vi "LineDetection-2Steps.vi"() -> ()   [LabVIEW 2014]
doc: "This example shows how to use the Edge Tool in NI Vision. The Edge Tool finds edges (or sharp transitions in the pixels values) along a given line or ROI profile. The Edge Tool is a precursor function to many of the gauging and inspection tasks. For example, the location of the edges found along a line profile across an object can interpreted as the boundaries of the object whose dimensions have to be measured for a gauging application or the presence of a crack in the surface of an object for an inspection application."
uses:
  <vilib>/vision/NI_Vision_Development_Module.lvlib
panel:
  in  "Process":u16(ring)=2 items=["Get First Edge", "Get First + Last Edge", "Get All Edges", "Get Best Edge"]
  in  "Scan Direction":u16
  in  "Step Size":u32=5
  in  "Edge Options":T1={"Edge Polarity"=0, "Kernel Size"=3, "Width"=5, "Minimum Edge Strength"=10.0, "Interpolation Type"=1, "Data Processing Method"=0} {"Data Processing Method" items=["Average", "Median"]; "Interpolation Type" items=["Zero Order"=0, "Bilinear"=1, "Bilinear Fixed"=4]; "Minimum Edge Strength" min=0.0 max=255.0 format="%.2g"; "Width" min=1 step=2; "Kernel Size" min=3 step=2; "Edge Polarity" items=["All Edges", "Rising Edges", "Falling Edges"]}
  out "Image":T2(plugin-control)
  in  "Stop":bool
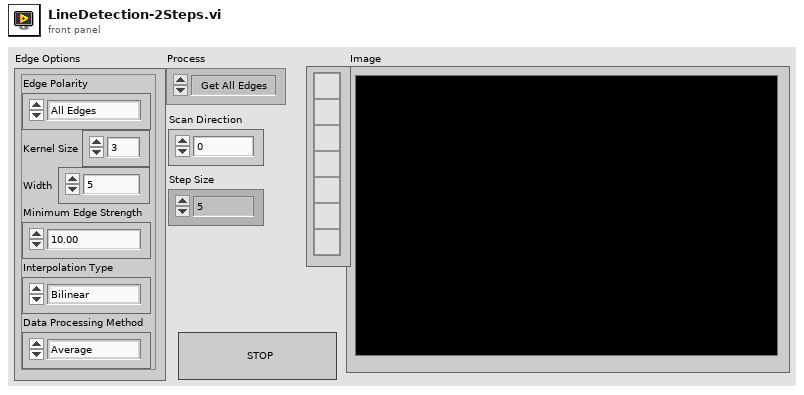
[diagram p1: front panel]
types:
  T1 = cluster{"Edge Polarity":u16, "Kernel Size":u32, "Width":u32, "Minimum Edge Strength":dbl, "Interpolation Type":u16, "Data Processing Method":u16}
  T2 = typedef "IMAQ Image.ctl" = refnum<image>
  T3 = typedef "IMAQ Circle" = cluster{"Center X":i32, "Center Y":i32, "Inner Radius":i32, "Outer Radius":i32, "Start Angle":dbl, "End Angle":dbl}
  T4 = typedef "ROI Descriptor" = cluster{"Global Rectangle":i32[], "Contours":cluster{"ID":enum32{"External", "Internal"}, "Type":u32, "Coordinates":i32[]}[]}
  T5 = cluster{"Edge Options":cluster{"Edge Polarity":u16, "Kernel Size":u32, "Width":u32, "Minimum Edge Strength":dbl, "Interpolation Type":u16, "Data Processing Method":u16}, "Step Size":u32, "Scan Direction":u16, "Process":u16}
  T6 = cluster{"Global Rectangle":i32[], "Contours":cluster{"Contour Type":u32, "ROI Type":u32, "Points":i32[]}[]}
  T7 = typedef "Edge New.ctl" = cluster{"Location (Pixel)":cluster{"X":sgl, "Y":sgl}, "Location (Real-World)":cluster{"X":sgl, "Y":sgl}, "Distance (Pixel)":dbl, "Distance (Real-World)":dbl, "Strength":dbl, "Noise":dbl, "Rising?":bool}
  T8 = cluster{"Point 1":cluster{"X":sgl, "Y":sgl}, "Point 2":cluster{"X":sgl, "Y":sgl}}
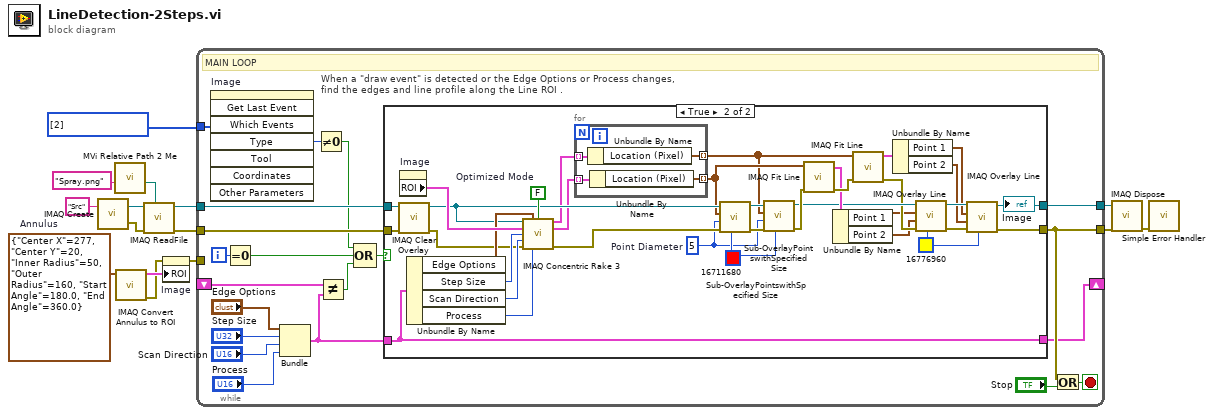
[diagram p0: block diagram]
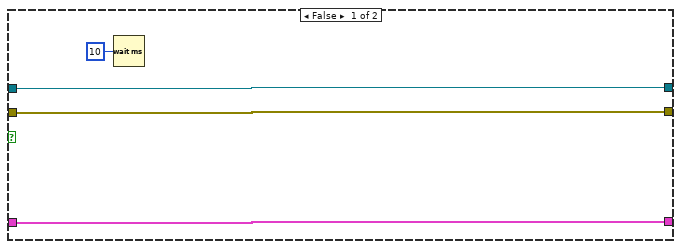
[diagram p2: hidden frame]
diagram:
  w1 = T3 {"Center X"=277, "Center Y"=20, "Inner Radius"=50, "Outer Radius"=160, "Start Angle"=180.0, "End Angle"=360.0}  # Annulus
  w7 = i32[] [2] items=["No  event", "Click event", "Draw event", "Move event", "Size event", "Scroll event", "Activate event", "Close event", "Double click event"] ("Events list (all)")
  n1 = call "IMAQ Create"("Image Name"="Src") -> ("New Image"=w14:T2, "error out"=w13:errorcluster)  [unwired: 4 in]
  n2 = call "MVi Relative Path 2 Me.vi"("Relative Path"="Spray.png" ("name or relative path")) -> ("Appended Dir"=w5:path)  [unwired: 5 in, 1 out]
  n3 = call "IMAQ Convert Annulus to ROI"("Annulus"=w1) -> ("error out"=w3:errorcluster, "ROI Descriptor"=w4:T4)  [unwired: 8 in]
  n4 = call "IMAQ ReadFile"("File Path"=w5, "error in (no error)"=w13, "Image"=w14) -> ("error out"=w8:errorcluster, "Image Out"=w9:T2)  [unwired: 4 in, 3 out]
  n5 = property on="Image" class="ImageControl"(error in=w3, "ROI"=w4) -> (error out=w2:errorcluster)  [unwired: 1 in, 1 out]
  n6 = while "MAIN LOOP" {
    tunnel: w9 -> [w34]
    tunnel: w8 -> [w35]
    tunnel: [w30] -> w12
    tunnel: [w31] -> w11
    tunnel: w7 -> [w29]
    shift-right: [w24] -> _
    shift-left: _ -> [w18]
    tunnel: w2 -> [_]
    i -> [w27]
    stop <- w32 stop-if-true
    # "When a \"draw event\" is detected or the Edge Options or Process changes, find the edges and line profile along the Line ROI ."
    # "MAIN LOOP"
    n7 = invoke on="Image" class="ImageControl" method="Get Last Event"("Which Events"=w29) -> ("Type"=w28:i32)  [unwired: 7 in, 7 out]
    n8 = Equal To 0?(x=w27) -> (x = 0?=w23:bool)
    n9 = Bundle("Edge Options"="Edge Options", "Step Size"="Step Size", "Scan Direction"="Scan Direction", "Process"="Process") -> (w19:T5)  [unwired: 1 in]
    n10 = Not Equal To 0?(x=w28) -> (x != 0?=w26:bool)
    n11 = Not Equal?(x=w18, y=w19) -> (x != y?=w17:bool)
    n12 = Compound Arithmetic op=OR(w26, w23, w17) -> (w25:bool)
    n13 = case shown="True" w25 {
      tunnel: w35 -> [w38 w72]
      tunnel: w34 -> [w39 w71]
      tunnel: [w39 w46] -> w31
      tunnel: [w38 w47] -> w30
      tunnel: [w36 w69] -> w24
      tunnel: w19 -> [w36 w69]
      frame False {
        n14 = Wait (ms)(milliseconds to wait=u32 10) -> ()  [unwired: 1 out]
      }
      frame True {
        w40 = u32 16776960 ("Color")
        w58 = u32 5  # Point Diameter
        w70 = FALSE  # Optimized Mode
        w59 = u32 16711680 ("Color")
        n15 = call "IMAQ Clear Overlay"("error in (no error)"=w72, "Image"=w71) -> ("error out"=w62:errorcluster, "Image Out"=w65:T2)  [unwired: 8 in]
        n16 = property on="Image" class="ImageControl"() -> ("ROI"=w73:T6)  [unwired: 2 in, 2 out]
        n17 = Unbundle By Name(w69) -> ("Edge Options"=w68:T1, "Step Size"=w67:u32, "Scan Direction"=w66:u16, "Process"=w57:u16)
        n18 = call "IMAQ Concentric Rake 3"("Image"=w65, "Edge Options"=w68, "Optimized Mode"=w70, "ROI Descriptor"=w73, "Step Size"=w67, "Scan Direction"=w66, "error in (no error)"=w62, "Process"=w57) -> ("First Edges"=w64:T7[], "Last Edges"=w63:T7[], "error out"=w74:errorcluster)  [unwired: 4 in, 1 out]
        n19 = for {
          tunnel: w64 -> [w77] mode=indexing
          tunnel: [w78] -> w53 mode=indexing
          tunnel: w63 -> [w76] mode=indexing
          tunnel: [w75] -> w55 mode=indexing
          n20 = Unbundle By Name(w77) -> ("Location (Pixel)"=w78:cluster{"X":sgl, "Y":sgl})
          n21 = Unbundle By Name(w76) -> ("Location (Pixel)"=w75:cluster{"X":sgl, "Y":sgl})
        }
        n22 = call "Sub-OverlayPointswithSpecified Size.vi"("Color"=w59, "error in"=w74, "Point Diameter (5)"=w58, "Points"=w55, "Image In"=w65) -> ("error out"=w61:errorcluster, "Image Out"=w60:T2)  [unwired: 5 in]
        n23 = call "Sub-OverlayPointswithSpecified Size.vi"("Color"=w59, "error in"=w61, "Point Diameter (5)"=w58, "Points"=w53, "Image In"=w60) -> ("error out"=w56:errorcluster, "Image Out"=w51:T2)  [unwired: 5 in]
        n24 = call "IMAQ Fit Line"("error in (no error)"=w56, "Points"=w55) -> ("error out"=w54:errorcluster, "Line Segment"=w52:T8)  [unwired: 4 in, 4 out]
        n25 = Unbundle By Name(w52) -> ("Point 1"=w45:cluster{"X":sgl, "Y":sgl}, "Point 2"=w44:cluster{"X":sgl, "Y":sgl})
        n26 = call "IMAQ Fit Line"("error in (no error)"=w54, "Points"=w53) -> ("error out"=w50:errorcluster, "Line Segment"=w43:T8)  [unwired: 4 in, 4 out]
        n27 = Unbundle By Name(w43) -> ("Point 1"=w41:cluster{"X":sgl, "Y":sgl}, "Point 2"=w42:cluster{"X":sgl, "Y":sgl})
        n28 = call "IMAQ Overlay Line"("Color"=w40, "error in (no error)"=w50, "End Point"=w44, "Start Point"=w45, "Image"=w51) -> ("error out"=w49:errorcluster, "Image Out"=w48:T2)  [unwired: 5 in]
        n29 = call "IMAQ Overlay Line"("Color"=w40, "error in (no error)"=w49, "End Point"=w42, "Start Point"=w41, "Image"=w48) -> ("error out"=w47:errorcluster, "Image Out"=w46:T2)  [unwired: 5 in]
        "Image" <- w46
      }
    }
    n30 = Or(x=w30, y="Stop") -> (x .or. y?=w32:bool)
  }
  n31 = call "IMAQ Dispose"("Image"=w11, "error in (no error)"=w12) -> ("error out"=w10:errorcluster)  [unwired: 4 in]
  n32 = call <vilib>:"Simple Error Handler.vi"("error in (no error)"=w10) -> ()  [unwired: 4 in, 5 out]
